vi "FVIR_LDO_Inficon.vi"(8 "error in":errorcluster, 10 "Remote IP Address":string="192.168.1.32", 11 "Message Queues":T1) -> (0 "error out":errorcluster)   [LabVIEW 2020]
uses:
  Message Queue/All Message Queues.ctl
  Message Queue/Message Cluster.ctl
  Drivers/Inficon Transmitter/Type Definitions/Inficon Data.ctl
  Message Queue/Enqueue Message (Single).vi
  <vilib>/NI/Modbus Library/API/Wrapper/Create TCP Master.vi
  <vilib>/NI/Modbus Library/API/Master/Modbus Master.lvclass
  Message Queue/Message Queue.lvlib
  <vilib>/NI/Modbus Library/API/Wrapper/API Main.lvlib
panel:
  out "Loop Count":i32
  # "NG Inficon: 192.168.1.32\nLP Inficon: 192.168.1.33"
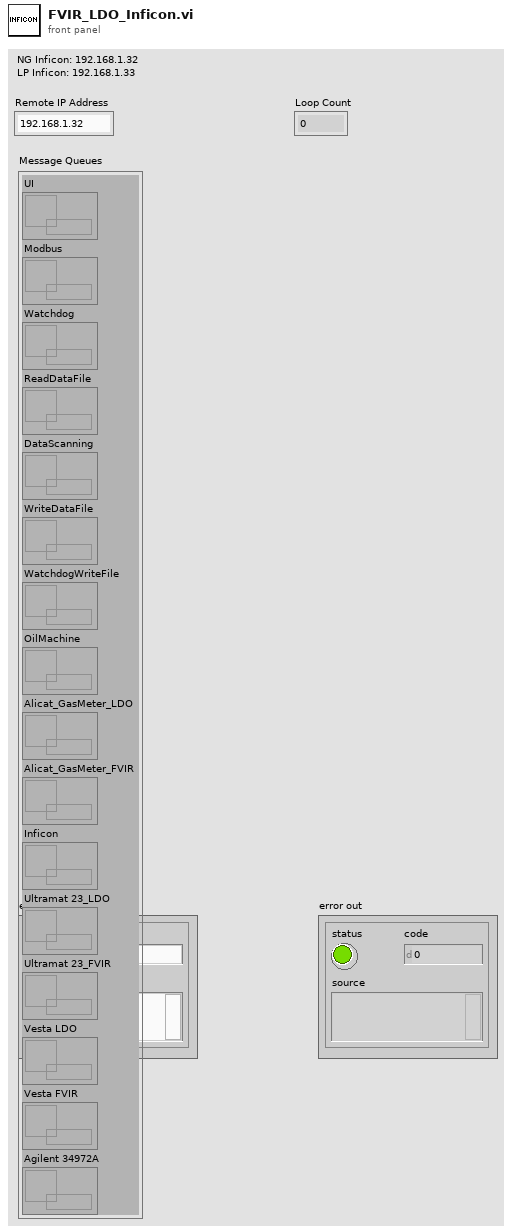
[diagram p1: front panel]
types:
  T1 = typedef "Message Queue.lvlib/All Message Queues.ctl" = cluster{"UI":refnum<queue>, "Modbus":refnum<queue>, "Watchdog":refnum<queue>, "ReadDataFile":refnum<queue>, "DataScanning":refnum<queue>, "WriteDataFile":refnum<queue>, "WatchdogWriteFile":refnum<queue>, "OilMachine":refnum<queue>, "Alicat_GasMeter_LDO":refnum<queue>, "Inficon":refnum<queue>, "Ultramat 23_LDO":refnum<queue>, "Alicat_GasMeter_FVIR":refnum<queue>, "Ultramat 23_FVIR":refnum<queue>, "Vesta LDO":refnum<queue>, "Vesta FVIR":refnum<queue>, "Agilent 34972A":refnum<queue>}
  T2 = typedef "Inficon Data.ctl" = cluster{"Gross Heating Value, Vol (Real, Dry)":dbl, "Nitrogen Component Normalized Mole % (Dry)":dbl, "Methane Component Normalized Mole % (Dry)":dbl, "Carbon Dioxide Component Normalized Mole % (Dry)":dbl, "Ethane Component Normalized Mole % (Dry)":dbl, "Propane Component Normalized Mole % (Dry)":dbl, "i-Pentane Component Normalized Mole % (Dry)":dbl, "i-Butane Component Normalized Mole % (Dry)":dbl, "n-Butane Component Normalized Mole % (Dry)":dbl, "n-Pentane Component Normalized Mole % (Dry)":dbl, "Hexane Component Normalized Mole % (Dry)":dbl, "Heptane Component Normalized Mole % (Dry)":dbl, "Gross Wobbe Index, Real(Dry)":dbl, "Relative Density, Real(Dry)":dbl, "Propylene Component Normalized Mole % (Dry)":dbl, "C4 Olefins Component Normalized Mole % (Dry)":dbl, "Water Component Normalized Mole % (Dry)":dbl}
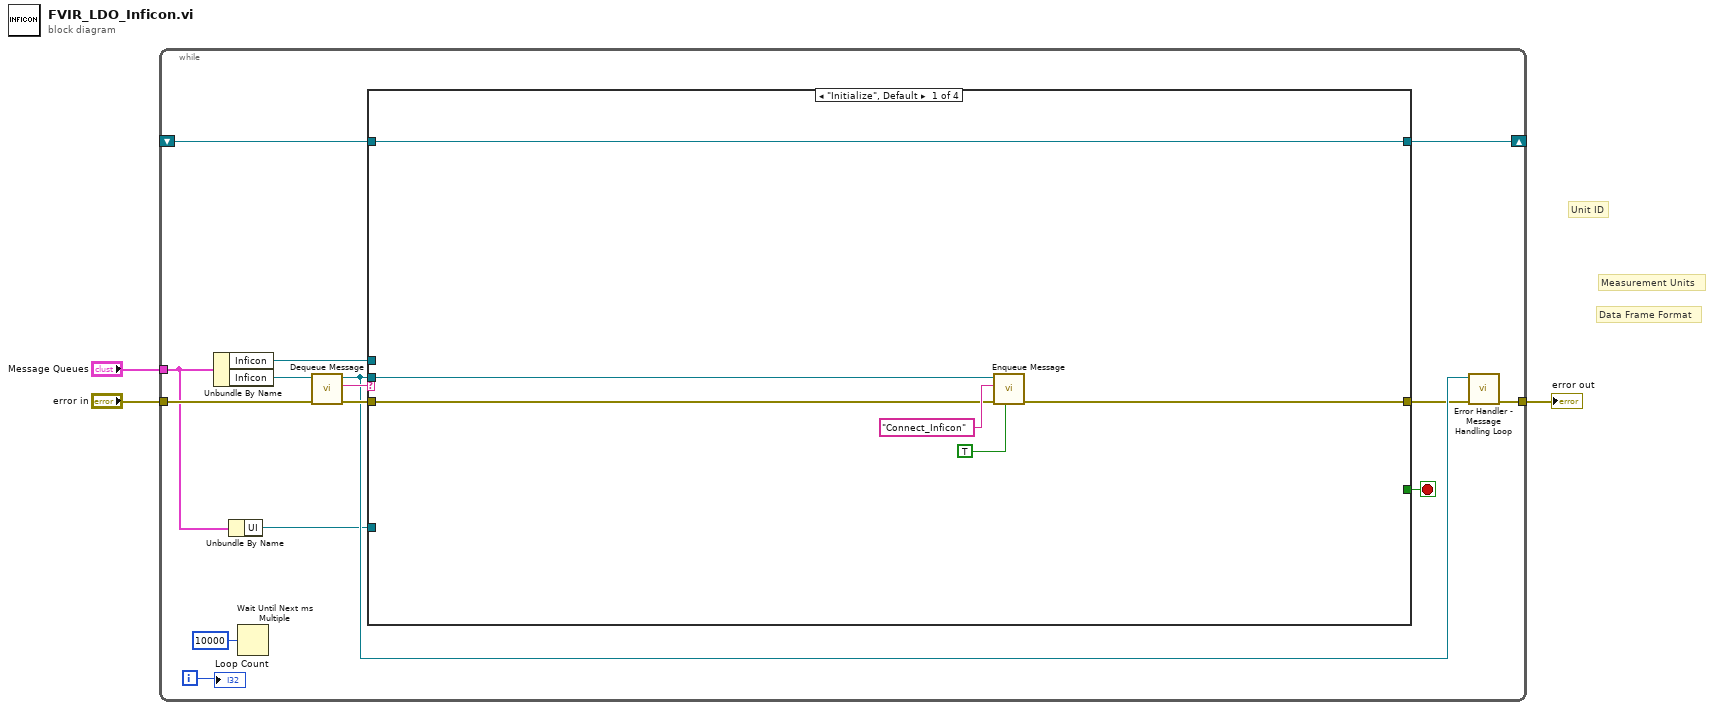
[diagram p0: block diagram]
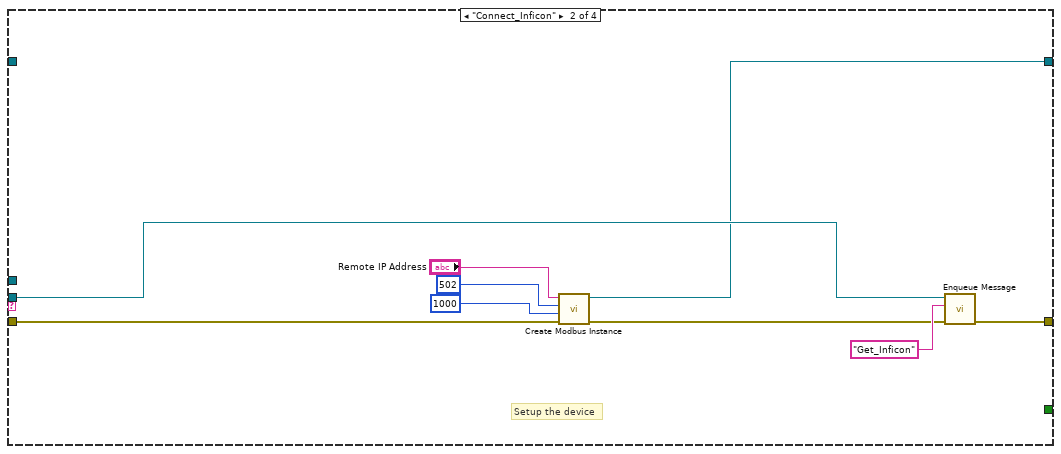
[diagram p2: hidden frame]
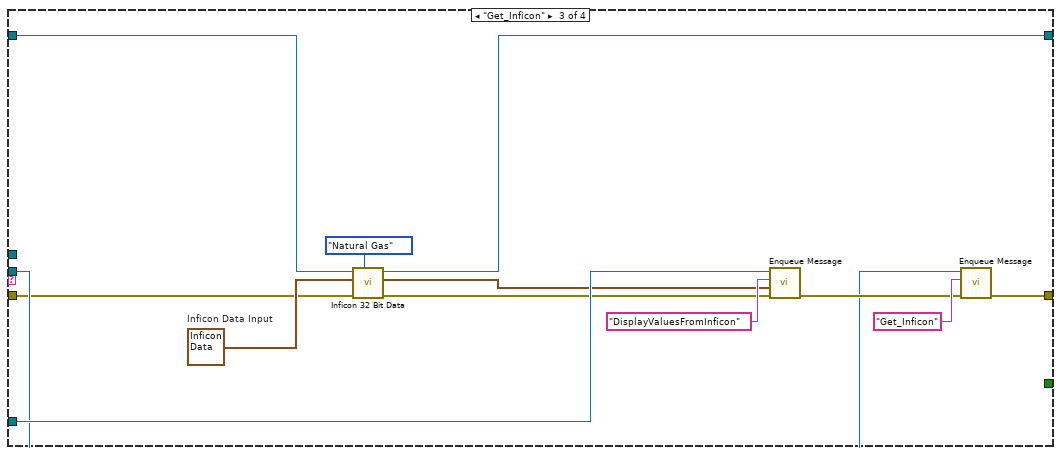
[diagram p3: hidden frame]
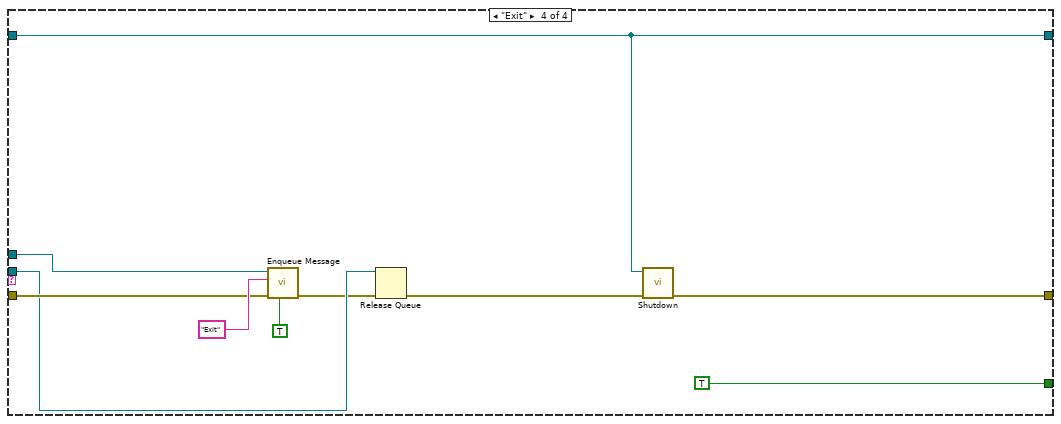
[diagram p4: hidden frame]
diagram:
  # "Unit ID"
  # "Data Frame Format"
  # "Measurement Units"
  n1 = while {
    tunnel: "Message Queues" -> [w8]
    tunnel: "error in" -> [w17]
    tunnel: [w11] -> w1
    shift-right: [w6] -> _
    shift-left: _ -> [w5]
    i -> [w4]
    stop <- w14 stop-if-true
    n2 = Unbundle By Name(w8) -> ("Inficon"=w13:refnum<queue>, "Inficon"=w18:refnum<queue>)
    n3 = Unbundle By Name(w8) -> ("UI"=w7:refnum<queue>)
    n4 = Wait Until Next ms Multiple(millisecond multiple=u32 10000) -> ()  [unwired: 1 out]
    n5 = call "Dequeue Message.vi"("error in (no error)"=w17, "Message Queue"=w18) -> ("error out"=w15:errorcluster, "Message"=w16:string, "dup Message Queue"=w12:refnum<queue>)  [unwired: 6 in, 1 out]
    n6 = case shown="\"Initialize\", Default" w16 {
      tunnel: w15 -> [w23 w26 w38 w52]
      tunnel: [w22 w32 w42 w48] -> w10
      tunnel: [_ _ _ TRUE] -> w14
      tunnel: w13 -> [_ _ _ w53]
      tunnel: w12 -> [w21 w31 w41 w51]
      tunnel: w7 -> [_ _ w45 _]
      tunnel: [w20 w25 w39 w47] -> w6
      tunnel: w5 -> [w20 _ w34 w47]
      frame "Initialize", Default {
        n7 = call-poly "Enqueue Message.vi"("Priority Message? (F)"=TRUE, "error in (no error)"=w23, "Message"="Connect_Inficon", "Message Queue"=w21) -> ("error out"=w22:errorcluster)  [unwired: 6 in, 1 out]
      }
      frame "Connect_Inficon" {
        # "Setup the device"
        n8 = call-poly <vilib>:"Create Modbus Instance.vi"("error in"=w26, "connect timeout ms"=1000, "port (502)"=u16 502, "address"="Remote IP Address") -> ("error out"=w27:errorcluster, "TCP master instance"=w25:refnum<class "Modbus Master.lvclass">)  [unwired: 6 in]
        n9 = call-poly "Enqueue Message.vi"("error in (no error)"=w27, "Message"="Get_Inficon", "Message Queue"=w31) -> ("error out"=w32:errorcluster)  [unwired: 7 in, 1 out]
      }
      frame "Get_Inficon" {
        w40 = T2 {"Gross Heating Value, Vol (Real, Dry)"=0.0, "Nitrogen Component Normalized Mole % (Dry)"=0.0, "Methane Component Normalized Mole % (Dry)"=0.0, "Carbon Dioxide Component Normalized Mole % (Dry)"=0.0, "Ethane Component Normalized Mole % (Dry)"=0.0, "Propane Component Normalized Mole % (Dry)"=0.0, "i-Pentane Component Normalized Mole % (Dry)"=0.0, "i-Butane Component Normalized Mole % (Dry)"=0.0, "n-Butane Component Normalized Mole % (Dry)"=0.0, "n-Pentane Component Normalized Mole % (Dry)"=0.0, "Hexane Component Normalized Mole % (Dry)"=0.0, "Heptane Component Normalized Mole % (Dry)"=0.0, "Gross Wobbe Index, Real(Dry)"=0.0, "Relative Density, Real(Dry)"=0.0, "Propylene Component Normalized Mole % (Dry)"=0.0, "C4 Olefins Component Normalized Mole % (Dry)"=0.0, "Water Component Normalized Mole % (Dry)"=0.0}  # Inficon Data Input
        n10 = call "Inficon 32 Bit Data.vi"("Gas Type"=enum16{"Natural Gas", "Propane Gas"}."Natural Gas", "Error In"=w38, "Inficon Data Input"=w40, "Modbus master in"=w34) -> ("Error Out"=w37:errorcluster, "Inficon Data Output"=w36:T2, "Modbus master out"=w39:refnum<class "Modbus Master.lvclass">)  [unwired: 4 in, 1 out]
        n11 = call-poly "Enqueue Message.vi"("error in (no error)"=w37, "Message Data"=w36, "Message"="DisplayValuesFromInficon", "Message Queue"=w45) -> ("error out"=w43:errorcluster)  [unwired: 6 in, 1 out]
        n12 = call-poly "Enqueue Message.vi"("error in (no error)"=w43, "Message"="Get_Inficon", "Message Queue"=w41) -> ("error out"=w42:errorcluster)  [unwired: 7 in, 1 out]
      }
      frame "Exit" {
        n13 = call-poly "Enqueue Message.vi"("Priority Message? (F)"=TRUE, "error in (no error)"=w52, "Message"="Exit", "Message Queue"=w53) -> ("error out"=w50:errorcluster)  [unwired: 6 in, 1 out]
        n14 = Release Queue(queue=w51, error in (no error)=w50) -> (error out=w49:errorcluster)  [unwired: 1 in, 2 out]
        n15 = call-dynamic "Shutdown.vi"("error in"=w49, "Modbus master in"=w47) -> ("error out"=w48:errorcluster)  [unwired: 9 in]
      }
    }
    n16 = call "Error Handler - Message Handling Loop.vi"("error in (no error)"=w10, "Message Queue"=w12) -> ("dup error in"=w11:errorcluster)  [unwired: 8 in, 1 out]
    "Loop Count" <- w4
  }
  "error out" <- w1
